vi "Get Device by Name.vi"(7 "Type":refnum<class "Device.lvclass">, 8 "error in (no error)":errorcluster, 10 "Device Name":string, 11 "HAL Manager in":refnum<class "HAL Manager.lvclass">) -> (0 "error out":errorcluster, 2 "Device":refnum<class "Device.lvclass">, 3 "HAL Manager out":refnum<class "HAL Manager.lvclass">)   [LabVIEW 2020, in "HAL.lvlib" / "HAL Manager.lvclass"]
uses:
  HAL Manager.lvclass
  Device/Device.lvclass
  HAL Manager.lvclass/HAL Manager.ctl
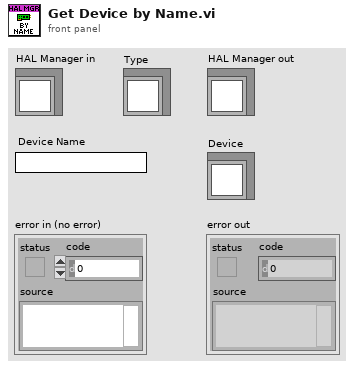
[diagram p1: front panel]
types:
  T1 = typedef "HAL.lvlib/HAL Manager.lvclass/Ref Data.ctl" = cluster{"Devices":refnum<class "Device.lvclass">[], "Type":string[], "Models":string[], "Name":string[]}
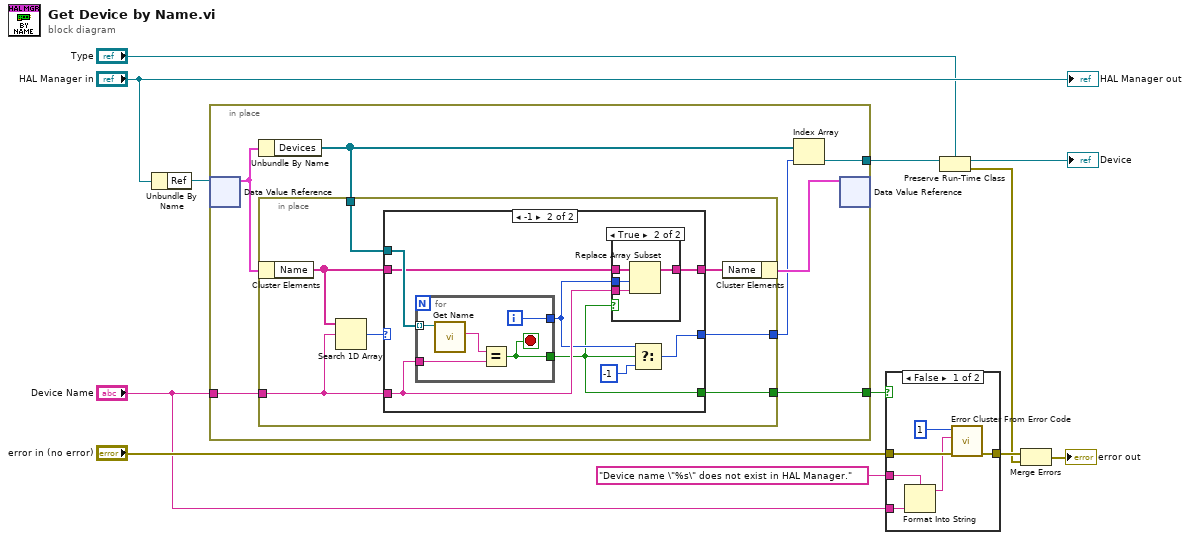
[diagram p0: block diagram]
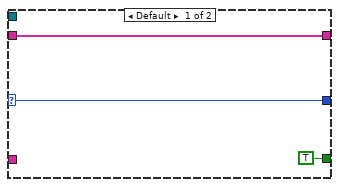
[diagram p3: hidden frame]
diagram:
  n1 = Unbundle By Name("HAL Manager in") -> ("Ref"=w12:refnum<data-value>)
  n2 = in-place {
    in-place-border: "Device Name" -> [w18]
    in-place-border: [w14] -> w10
    in-place-border: [w13] -> w6
    n3 = in-place-dvr #1(w12) -> (w19:T1)  [unwired: 1 out]
    n4 = Unbundle By Name(w19) -> ("Devices"=w16:refnum<class "Device.lvclass">[])
    n5 = in-place {
      in-place-border: w18 -> [w24]
      in-place-border: w16 -> [w25]
      in-place-border: [w21] -> w15
      in-place-border: [w20] -> w13
      n6 = in-place-cluster #2(w19) -> ("Name"=w23:string[])
      n7 = Search 1D Array(1D array=w23, element=w24) -> (index of element=w26:i32)  [unwired: 1 in]
      n8 = case shown="-1" w26 {
        selector: w26 -> [w28 _]
        tunnel: w25 -> [_ w37]
        tunnel: w24 -> [_ w35]
        tunnel: w23 -> [w29 w36]
        tunnel: [w29 w34] -> w22
        tunnel: [w28 w32] -> w21
        tunnel: [TRUE w30] -> w20
        frame Default {
        }
        frame -1 {
          n9 = for {
            tunnel: w37 -> [w47] mode=indexing
            tunnel: w35 -> [w46]
            tunnel: [w44] -> w30
            tunnel: [w43] -> w33
            i -> [w43]
            stop <- w44 stop-if-true
            n10 = call "Get Name.vi"("Device in"=w47) -> ("Name"=w45:string)  [unwired: 8 in, 2 out]
            n11 = Equal?(x=w45, y=w46) -> (x = y?=w44:bool)
          }
          n12 = case shown="True" w30 {
            tunnel: w36 -> [w38 w42]
            tunnel: w35 -> [_ w41]
            tunnel: w33 -> [_ w40]
            tunnel: [w38 w39] -> w34
            frame False {
            }
            frame True {
              n13 = Replace Array Subset(array=w42, new element=w41, index=w40) -> (w39:string[])
            }
          }
          n14 = Select(t=w33, s=w30, f=-1) -> (s? t:f=w32:i32)
        }
      }
      n15 = in-place-cluster #2("Name"=w22) -> (w17:T1)
    }
    n16 = Index Array(array=w16, index=w15) -> (element=w14:refnum<class "Device.lvclass">)
    n17 = in-place-dvr #1(w17) -> ()  [unwired: 2 out]
  }
  n18 = case shown="False" w6 {
    tunnel: "error in (no error)" -> [w53 w54]
    tunnel: [w51 w54] -> w5
    tunnel: "Device name \"%s\" does not exist in HAL Manager." -> [w49 _]
    tunnel: "Device Name" -> [w50 _]
    frame False {
      n19 = Format Into String(format string=w49, w50) -> (resulting string=w48:string)  [unwired: 2 in, 1 out]
      n20 = call <vilib>:"Error Cluster From Error Code.vi"("error in (no error)"=w53, "error message (\"\")"=w48, "error code (0)"=1) -> ("error out"=w51:errorcluster)  [unwired: 6 in]
    }
    frame True {
    }
  }
  n21 = Preserve Run-Time Class(object in=w10, 2:"Type") -> (object out=→"Device":refnum<class "Device.lvclass">, error out=w4:errorcluster)  [unwired: 1 in]
  n22 = Merge Errors(w5, w4) -> (→"error out":errorcluster)
  "HAL Manager out" <- "HAL Manager in"
